vi "example_04_busy_wait.vi"() -> ()   [LabVIEW 2015, in "lv-dialog.lvlib" / "v1.lvlib"]
uses:
  v1.lvlib
  public/_controls/selection.ctl
  public/class/v1.lvclass
panel:
  in  "milliseconds to wait":u32=1000
  in  "outer_color":u32(colorbox)=6618880
  in  "inner_color":u32(colorbox)=16711680
  in  "wait_s":dbl=5.0 format="%#_13g"
  in  "dialog_text":string="Wait for the Process"
  out "error":errorcluster
  out "dialog_selection":T1
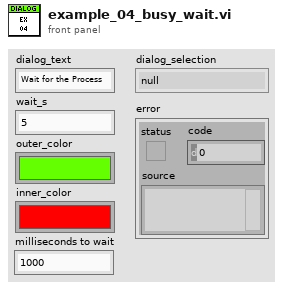
[diagram p1: front panel]
types:
  T1 = typedef "lv-dialog.lvlib/v1.lvlib/selection.ctl" = enum16{"null", "panel_closed", "button_1", "button_2", "button_3", "cancelled"}
  T2 = cluster{"dialog_text":string, "wait_s":dbl, "inner_color":u32, "outer_color":u32, "Event Registration Refnum":refnum<event-registration>}
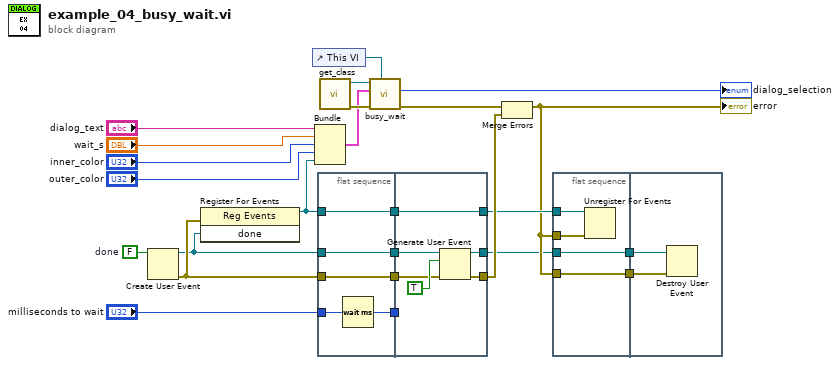
[diagram p0: block diagram]
diagram:
  w15 = FALSE  # done
  n1 = Create User Event(user event datatype=w15) -> (user event=w12:refnum<user-event>, error out=w25:errorcluster)  [unwired: 1 in]
  n2 = register-events(error in=w25, w12) -> (reference out=w9:refnum<event-registration>)  [unwired: 1 in, 1 out]
  n3 = control-ref of="This VI"() -> (w24:refnum<vi>)
  n4 = Bundle("dialog_text"="dialog_text", "wait_s"="wait_s", "inner_color"="inner_color", "outer_color"="outer_color", "Event Registration Refnum"=w9) -> (w16:T2)  [unwired: 1 in]
  n5 = flat-sequence {
    tunnel: w12 -> [w29]
    tunnel: [w29] -> w14
    tunnel: "milliseconds to wait" -> [w26]
    tunnel: w25 -> [w28]
    tunnel: [w28] -> w10
    tunnel: w9 -> [w27]
    tunnel: [w27] -> w8
    tunnel: [w26] -> w7
    tunnel: w14 -> [w35]
    tunnel: w10 -> [w31]
    tunnel: w8 -> [w30]
    tunnel: w7 -> [_]
    tunnel: [w33] -> w6
    tunnel: [w32] -> w2
    tunnel: [w30] -> w5
    frame #0 {
      n6 = Wait (ms)(milliseconds to wait=w26) -> ()  [unwired: 1 out]
    }
    frame #1 {
      n7 = Generate User Event(user event=w35, event data cluster=TRUE, error in=w31) -> (user event out=w32:refnum<user-event>, error out=w33:errorcluster)  [unwired: 1 in]
    }
  }
  n8 = call "get_class.vi"() -> ("error out"=w21:errorcluster, "class"=w22:refnum<class "v1.lvclass">)  [unwired: 10 in]
  n9 = call-dynamic "busy_wait.vi"("caller"=w24, "error in (no error)"=w21, "configuration"=w16, "v1 in"=w22) -> ("error out"=w11:errorcluster, "dialog_selection"=→"dialog_selection":T1)  [unwired: 5 in, 1 out]
  n10 = Merge Errors(w11, w6) -> (w3:errorcluster)
  "error" <- w3
  n11 = flat-sequence {
    tunnel: w5 -> [w37]
    tunnel: w3 -> [w39]
    tunnel: [w39] -> w4
    tunnel: w3 -> [w38]
    tunnel: w2 -> [w36]
    tunnel: [w36] -> w1
    tunnel: w4 -> [w41]
    tunnel: w1 -> [w40]
    frame #0 {
      n12 = Unregister For Events(event registration refnum=w37, error in=w38) -> ()  [unwired: 1 out]
    }
    frame #1 {
      n13 = Destroy User Event(user event=w40, error in=w41) -> ()  [unwired: 1 out]
    }
  }
